vi "Init Ping Packet.vi"(5 "Data Size in Bytes (32)":i32=32, 7 "Sequence Number":u16, 8 "Error In":errorcluster, 10 "ProcessID (0=Get PID)":u32 format="%04x") -> (0 "Error Out":errorcluster, 2 "ProcessID":u32 format="%04x", 3 "Output Packet":u8[](array[numeric]) format="%02x")   [LabVIEW 2018]
uses:
  kernel32.dll
panel:
  # "U32"
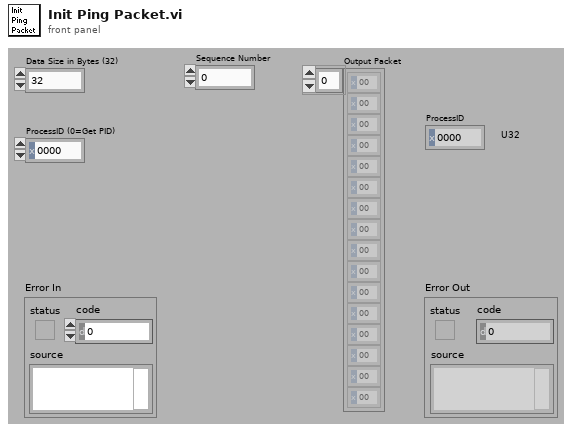
[diagram p1: front panel]
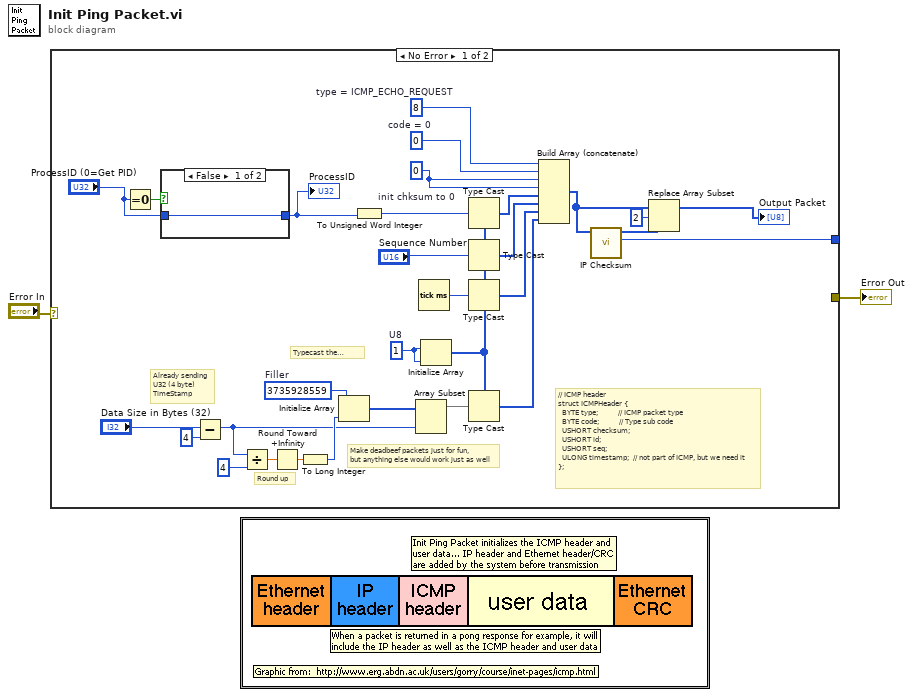
[diagram p0: block diagram]
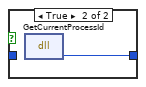
[diagram p2: hidden frame]
diagram:
  n1 = case shown="No Error" "Error In" {
    selector: "Error In" -> [_ w35]
    tunnel: [_ w35] -> w1
    tunnel: [w21 _] -> _
    frame No Error {
      w24 = u8 1  # U8
      w30 = u8 0  # init chksum to 0
      w31 = u8 0  # code = 0
      w32 = u8 8  # type = ICMP_ECHO_REQUEST
      w14 = u32 3735928559  # Filler
      # "Already sending \nU32 (4 byte)\nTimeStamp"
      # "Make deadbeef packets just for fun,\nbut anything else would work just as well"
      # "Round up"
      # "Typecast the results"
      # "// ICMP header\nstruct ICMPHeader {\n  BYTE type;          // ICMP packet type\n  BYTE code;          // Type sub code\n  USHORT checksum;\n  USHORT id;\n  USHORT seq;\n  ULONG timestamp;  // not part of ICMP, but we need it\n};"
      n2 = Equal To 0?(x="ProcessID (0=Get PID)") -> (x = 0?=w13:bool)
      n3 = case shown="False" w13 {
        tunnel: [w33 w34] -> w26
        tunnel: "ProcessID (0=Get PID)" -> [w33 _]
        frame False {
        }
        frame True {
          n4 = dll-call lib="kernel32.dll" fn="GetCurrentProcessId" label="GetCurrentProcessID()"() -> (w34:u32)  [unwired: 3 in, 2 out]
        }
      }
      "ProcessID" <- w26
      n5 = Subtract(x="Data Size in Bytes (32)", y=4) -> (x-y=w3:i32)
      n6 = Divide(x=w3, y=4) -> (x/y=w19:dbl)
      n7 = Round Toward +Infinity(x=w19) -> (ceil(x): smallest int >= x=w18:dbl)
      n8 = To Long Integer(number=w18) -> (32bit integer=w17:i32)
      n9 = Initialize Array(w14, w17) -> (w16:u32[])
      n10 = To Unsigned Word Integer(number=w26) -> (unsigned 16bit integer=w6:u16)
      n11 = Array Subset "Array Subset"(array=w16, length=w3) -> (w15:u32[])  [unwired: 1 in]
      n12 = Tick Count (ms)() -> (millisecond timer value=w22:u32)
      n13 = Initialize Array(w24, w24) -> (w7:u8[])
      n14 = Type Cast(type=w7, x=w6) -> (*(type *) &x=w8:u8[])
      n15 = Type Cast(type=w7, x="Sequence Number") -> (*(type *) &x=w9:u8[])
      n16 = Type Cast(type=w7, x=w22) -> (*(type *) &x=w11:u8[])
      n17 = Type Cast(type=w7, x=w15) -> (*(type *) &x=w25:u8[])
      n18 = Build Array (concatenate) "Build Array"(w32, w31, w30, w30, w8, w9, w11, w25) -> (w29:u8[])
      n19 = call "IP Checksum.vi"("Packet (U8)"=w29) -> ("cksum (U16)"=w21:u16, "cksum (U8 Array)"=w27:u8[])  [unwired: 7 in, 2 out]
      n20 = Replace Array Subset "Replace Array Subset"(array=w29, new element=w27, index=2) -> (→"Output Packet":u8[])
    }
    frame Error {
    }
  }
  "Error Out" <- w1
